vi "Drive Cycle Engine Request State ERD.vi"(0 "GEA2 Reference In":refnum<k24>, 1 "GEA Inputs":T2 {"Destination" format="%.0x"; "Source" format="%.0x"}, 2 "Standalone?":bool, 7 "Cycle ID":u8, 9 "Drive Cycle Engine Request State":T1=enum."Select", 11 "Error In":errorcluster) -> (4 "GEA2 Reference Out":refnum<k24>, 15 "Error Out":errorcluster)   [LabVIEW 2018, in "TLMB.lvlib"]
doc: "This vi can be used to update the MC cycle engine state with the requested values."
uses:
  Projects/TLMB.lvlib
  D:/Common/LabVIEW GEA2 Toolkit/source/GEA3 DLL Source/GeaCommunication.dll
  Common/LabVIEW GEA2 Toolkit/source/GEA3 DLL Source/GeaCommunication.dll
  Common/LabVIEW GEA2 Toolkit/GEA3/type defs/Source_Destination.ctl
  type defs/Drive Cycle Engine Request State.ctl
  Common/LabVIEW GEA2 Toolkit/GEA3/type defs/ERD Write Data In.ctl
  Common/LabVIEW GEA2 Toolkit/GEA3/type defs/Data Type.ctl
  C:/Users/iallatyp/Desktop/New folder/GEA3/library/GEA2_Toolkit.lvlib
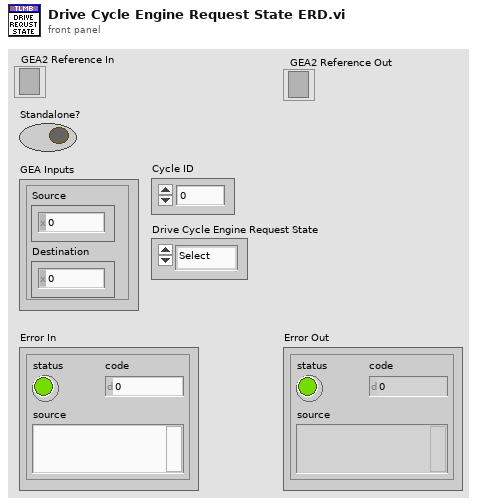
[diagram p1: front panel]
types:
  T1 = typedef "TLMB.lvlib/Drive Cycle Engine Request State.ctl" = enum16{"Start", "Stop", "Pause", "Resume", "Select"}
  T2 = typedef "GEA2_Toolkit.lvlib/Source_Destination.ctl" = cluster{"Source":u8, "Destination":u8}
  T3 = typedef "GEA2_Toolkit.lvlib/ERD Write Data In.ctl" = cluster{"ERD Number":u16, "Data Type":T4, "Data":string}
  T4 = typedef "GEA2_Toolkit.lvlib/Data Type.ctl" = enum16{"string", "boolean", "uint8_t", "uint16_t", "uint32_t", "uint64_t", "int8_t", "int16_t", "int32_t", "int64_t"}
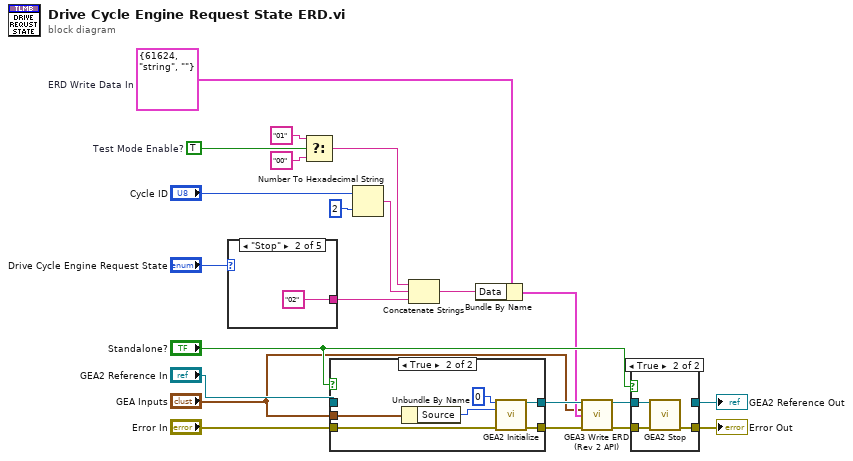
[diagram p0: block diagram]
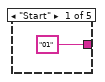
[diagram p2: hidden frame]
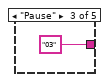
[diagram p3: hidden frame]
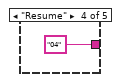
[diagram p4: hidden frame]
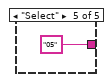
[diagram p5: hidden frame]
diagram:
  w11 = TRUE  # Test Mode Enable?
  w22 = T3 {"ERD Number"=61624, "Data Type"=enum."string", "Data"=""}  # ERD Write Data In
  n1 = case shown="\"Stop\"" "Drive Cycle Engine Request State" {
    tunnel: ["01" ("Message") "02" ("Message") "03" ("Message") "04" ("Message") "05" ("Message")] -> w12
    frame "Start" {
    }
    frame "Stop" {
    }
    frame "Pause" {
    }
    frame "Resume" {
    }
    frame "Select" {
    }
  }
  n2 = Select(t="01" ("Message"), s=w11, f="00" ("Message")) -> (s? t:f=w14:string)
  n3 = case shown="True" "Standalone?" {
    tunnel: "Error In" -> [w28 w35]
    tunnel: [w28 w34] -> w5
    tunnel: "GEA2 Reference In" -> [w29 _]
    tunnel: [w29 w33] -> w7
    tunnel: "GEA Inputs" -> [_ w31]
    frame False {
    }
    frame True {
      n4 = Unbundle By Name(w31) -> ("Source"=w32:u8)
      n5 = call "GEA2 Initialize.vi"("Board Index"=0, "Source Address"=w32, "error in"=w35) -> ("GEA2 Reference Out"=w33:refnum<k24>, "error out"=w34:errorcluster)  [unwired: 10 in, 1 out]
    }
  }
  n6 = Number To Hexadecimal String(1:i16 2 ("width (-)"), 2:"Cycle ID") -> (0:w13:string)
  n7 = Concatenate Strings(w14, w13, w12) -> (w8:string)
  n8 = Bundle By Name(cluster=w22, "Data"=w8) -> (w3:T3)
  n9 = call "GEA3 Write ERD (Rev 2 API).vi"("GEA2 Reference In"=w7, "GEA Inputs"="GEA Inputs", "ERD Write Data In"=w3, "Error In"=w5) -> ("GEA2 Reference Out"=w6:refnum<k24>, "Error Out"=w4:errorcluster)  [unwired: 9 in, 1 out]
  n10 = case shown="True" "Standalone?" {
    tunnel: [w36 w40] -> w21
    tunnel: w6 -> [w37 w39]
    tunnel: w4 -> [w36 w38]
    tunnel: [w37 _] -> w1
    frame False {
    }
    frame True {
      n11 = call "GEA2 Stop.vi"("GEA2 Reference In"=w39, "Error In"=w38) -> ("Error Out"=w40:errorcluster)  [unwired: 13 in]
    }
  }
  "Error Out" <- w21
  "GEA2 Reference Out" <- w1
